vi "Build Combos.vi"(11 "updated tags":T2(array[cluster])) -> (3 "Array":T1(array[cluster]))   [LabVIEW 2025]
panel:
  in  "index":i32=11
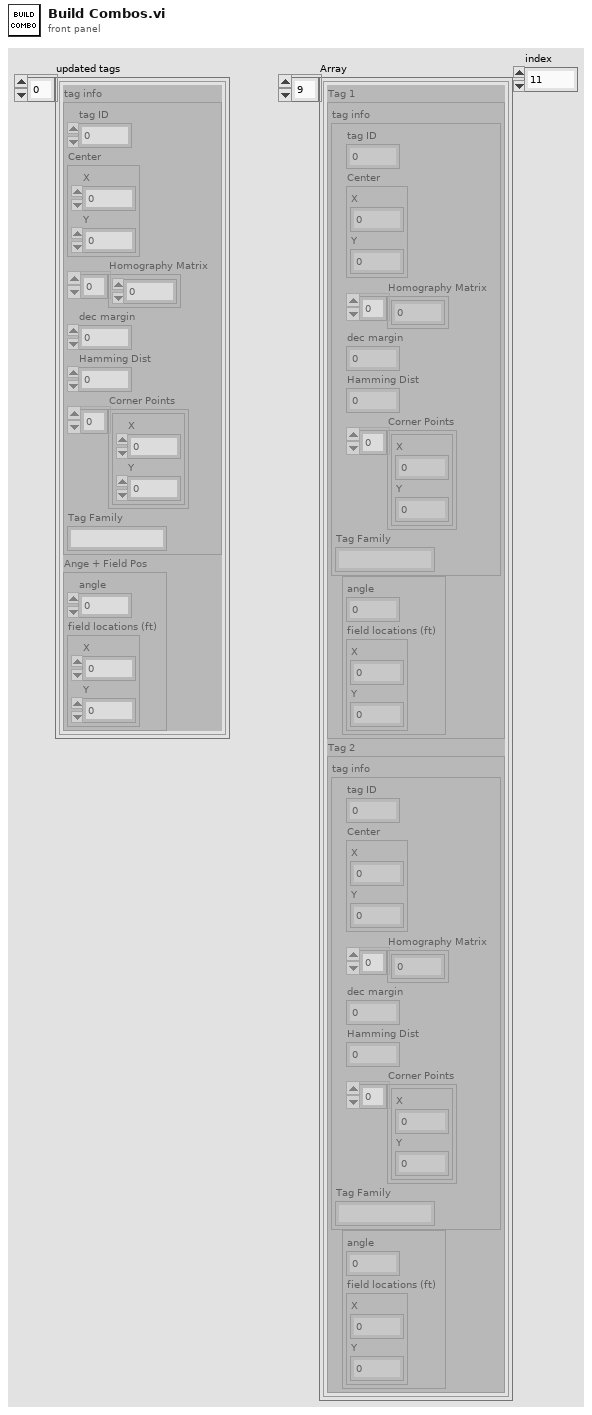
[diagram p1: front panel]
types:
  T1 = cluster{"Tag 1":cluster{"tag info":cluster{"tag ID":i32, "Center":cluster{"X":dbl, "Y":dbl}, "Homography Matrix":dbl[], "dec margin":dbl, "Hamming Dist":i32, "Corner Points":cluster{"X":dbl, "Y":dbl}[], "Tag Family":string}, cluster{"angle":dbl, "field locations (ft)":cluster{"X":dbl, "Y":dbl}}}, "Tag 2":cluster{"tag info":cluster{"tag ID":i32, "Center":cluster{"X":dbl, "Y":dbl}, "Homography Matrix":dbl[], "dec margin":dbl, "Hamming Dist":i32, "Corner Points":cluster{"X":dbl, "Y":dbl}[], "Tag Family":string}, cluster{"angle":dbl, "field locations (ft)":cluster{"X":dbl, "Y":dbl}}}}[]
  T2 = cluster{"tag info":cluster{"tag ID":i32, "Center":cluster{"X":dbl, "Y":dbl}, "Homography Matrix":dbl[], "dec margin":dbl, "Hamming Dist":i32, "Corner Points":cluster{"X":dbl, "Y":dbl}[], "Tag Family":string}, "Ange + Field Pos":cluster{"angle":dbl, "field locations (ft)":cluster{"X":dbl, "Y":dbl}}}[]
  T3 = cluster{"Tag 1":cluster{"tag info":cluster{"tag ID":i32, "Center":cluster{"X":dbl, "Y":dbl}, "Homography Matrix":dbl[], "dec margin":dbl, "Hamming Dist":i32, "Corner Points":cluster{"X":dbl, "Y":dbl}[], "Tag Family":string}, cluster{"angle":dbl, "field locations (ft)":cluster{"X":dbl, "Y":dbl}}}, "Tag 2":cluster{"tag info":cluster{"tag ID":i32, "Center":cluster{"X":dbl, "Y":dbl}, "Homography Matrix":dbl[], "dec margin":dbl, "Hamming Dist":i32, "Corner Points":cluster{"X":dbl, "Y":dbl}[], "Tag Family":string}, cluster{"angle":dbl, "field locations (ft)":cluster{"X":dbl, "Y":dbl}}}}
  T4 = cluster{"tag info":cluster{"tag ID":i32, "Center":cluster{"X":dbl, "Y":dbl}, "Homography Matrix":dbl[], "dec margin":dbl, "Hamming Dist":i32, "Corner Points":cluster{"X":dbl, "Y":dbl}[], "Tag Family":string}, "Ange + Field Pos":cluster{"angle":dbl, "field locations (ft)":cluster{"X":dbl, "Y":dbl}}}
  T5 = cluster{"tag info":cluster{"tag ID":i32, "Center":cluster{"X":dbl, "Y":dbl}, "Homography Matrix":dbl[], "dec margin":dbl, "Hamming Dist":i32, "Corner Points":cluster{"X":dbl, "Y":dbl}[], "Tag Family":string}, cluster{"angle":dbl, "field locations (ft)":cluster{"X":dbl, "Y":dbl}}}[]
  T6 = cluster{"[0]":cluster{"tag info":cluster{"tag ID":i32, "Center":cluster{"X":dbl, "Y":dbl}, "Homography Matrix":dbl[], "dec margin":dbl, "Hamming Dist":i32, "Corner Points":cluster{"X":dbl, "Y":dbl}[], "Tag Family":string}, cluster{"angle":dbl, "field locations (ft)":cluster{"X":dbl, "Y":dbl}}}, "[1]":cluster{"tag info":cluster{"tag ID":i32, "Center":cluster{"X":dbl, "Y":dbl}, "Homography Matrix":dbl[], "dec margin":dbl, "Hamming Dist":i32, "Corner Points":cluster{"X":dbl, "Y":dbl}[], "Tag Family":string}, cluster{"angle":dbl, "field locations (ft)":cluster{"X":dbl, "Y":dbl}}}}
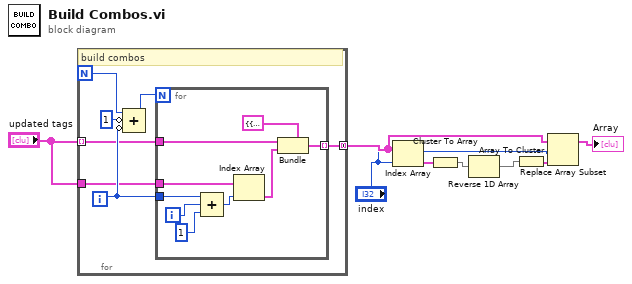
[diagram p0: block diagram]
diagram:
  n1 = for {
    N -> [w9]
    tunnel: [w15] -> w4 mode=concatenating
    tunnel: "updated tags" -> [w11] mode=indexing
    tunnel: "updated tags" -> [w10]
    i -> [w13]
    # "build combos"
    n2 = Compound Arithmetic op=ADD(w9, invert 1 ("value"), invert w13) -> (w14:i32)
    n3 = for {
      N: w14 -> [_]
      tunnel: w13 -> [w22]
      tunnel: [w19] -> w15 mode=indexing
      tunnel: w11 -> [w18]
      tunnel: w10 -> [w17]
      i -> [w21]
      n4 = Compound Arithmetic op=ADD(w22, w21, 1 ("value")) -> (w23:i32)
      n5 = Index Array(array=w17, index=w23) -> (element=w24:T4)
      n6 = Bundle(cluster=T3 {"Tag 1"={"tag info"={"tag ID"=0, "Center"={"X"=0.0, "Y"=0.0}, "Homography Matrix"=[], "dec margin"=0.0, "Hamming Dist"=0, "Corner Points"=[], "Tag Family"=""}, {"angle"=0.0, "field locations (ft)"={"X"=0.0, "Y"=0.0}}}, "Tag 2"={"tag info"={"tag ID"=0, "Center"={"X"=0.0, "Y"=0.0}, "Homography Matrix"=[], "dec margin"=0.0, "Hamming Dist"=0, "Corner Points"=[], "Tag Family"=""}, {"angle"=0.0, "field locations (ft)"={"X"=0.0, "Y"=0.0}}}} ("Combo"), "Tag 1"=w18, "Tag 2"=w24) -> (w19:T3)
    }
  }
  n7 = Index Array(array=w4, index="index") -> (element=w7:T3)
  n8 = Cluster To Array(cluster=w7) -> (array=w6:T5)
  n9 = Reverse 1D Array(array=w6) -> (reversed array=w5:T5)
  n10 = Array To Cluster(array=w5) -> (cluster=w3:T6)
  n11 = Replace Array Subset(array=w4, new element=w3, index="index") -> (→"Array":T1)
